vi "Create Arm Constants.vi"(1 "error in":errorcluster, 2 "localConstantSpreadSheet":string[][](array[string]), 3 "robotID":string) -> (0 "error out":errorcluster)   [LabVIEW 2020]
uses:
  2023 Robot Global Data.vi
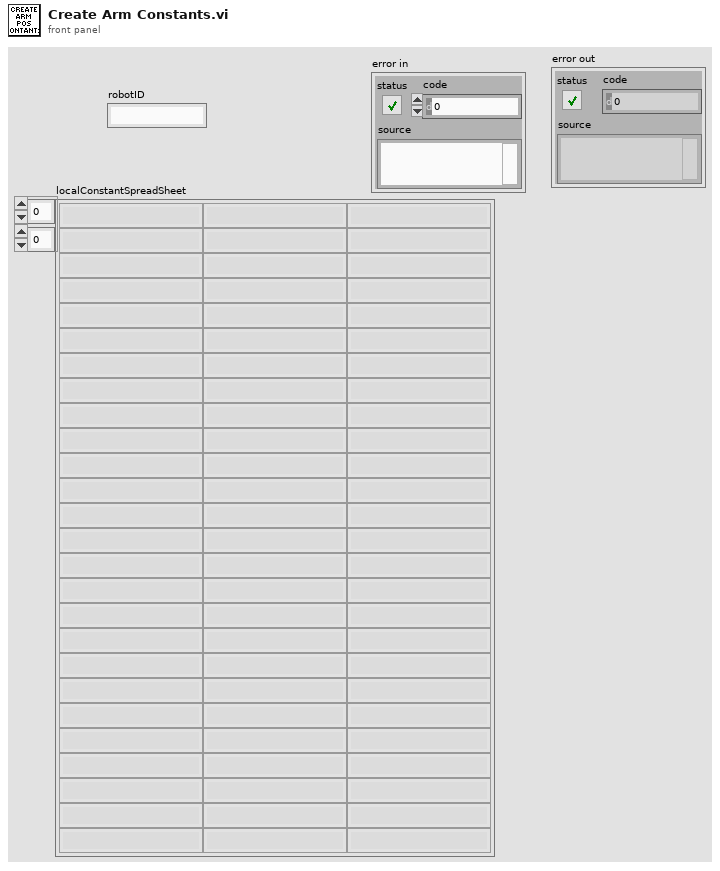
[diagram p1: front panel]
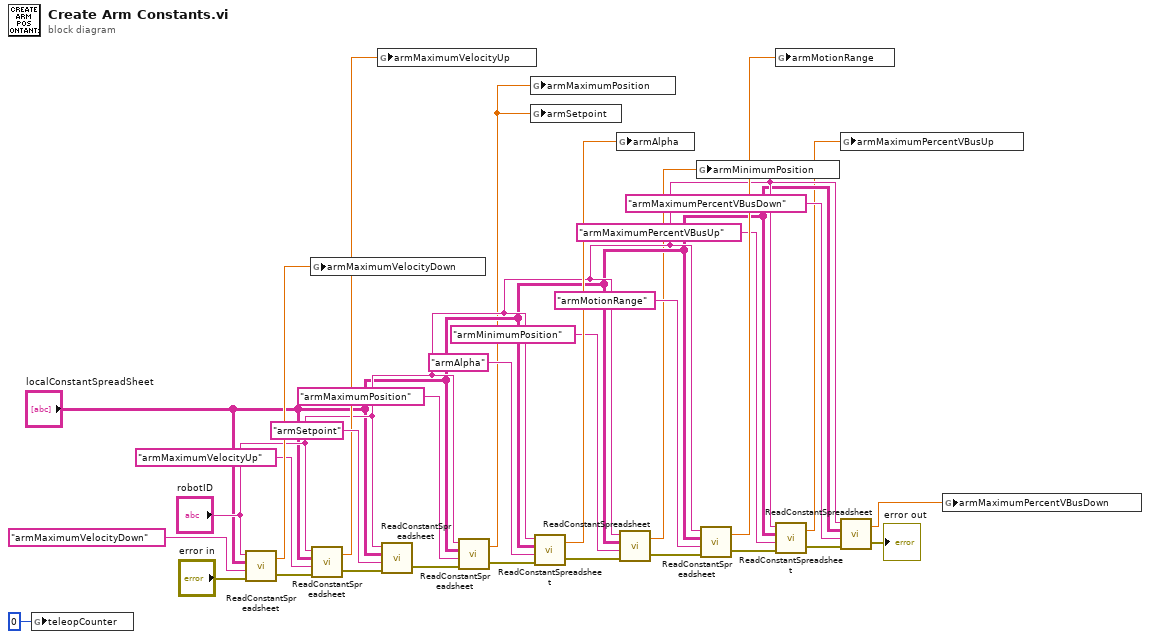
[diagram p0: block diagram]
diagram:
  n1 = global write "2023 Robot Global Data.vi" "teleopCounter"(0 ("teleopCounter")) -> ()
  n2 = call "ReadConstantSpreadsheet.vi"("error in"="error in", "Constant"="armMaximumVelocityDown", "2023ConstantSpreadSheet"="localConstantSpreadSheet", "Robot ID"="robotID") -> ("error out"=w13:errorcluster, "Constant Value"=w28:dbl)
  n3 = global write "2023 Robot Global Data.vi" "armMaximumVelocityDown"(w28) -> ()
  n4 = call "ReadConstantSpreadsheet.vi"("error in"=w13, "Constant"="armMaximumVelocityUp", "2023ConstantSpreadSheet"="localConstantSpreadSheet", "Robot ID"="robotID") -> ("error out"=w12:errorcluster, "Constant Value"=w11:dbl)
  n5 = global write "2023 Robot Global Data.vi" "armMaximumVelocityUp"(w11) -> ()
  n6 = call "ReadConstantSpreadsheet.vi"("error in"=w12, "Constant"="armSetpoint", "2023ConstantSpreadSheet"="localConstantSpreadSheet", "Robot ID"="robotID") -> ("error out"=w5:errorcluster)  [unwired: 1 out]
  n7 = call "ReadConstantSpreadsheet.vi"("error in"=w5, "Constant"="armMaximumPosition", "2023ConstantSpreadSheet"="localConstantSpreadSheet", "Robot ID"="robotID") -> ("error out"=w20:errorcluster, "Constant Value"=w2:dbl)
  n8 = global write "2023 Robot Global Data.vi" "armMaximumPosition"(w2) -> ()
  n9 = global write "2023 Robot Global Data.vi" "armSetpoint"(w2) -> ()
  n10 = call "ReadConstantSpreadsheet.vi"("error in"=w20, "Constant"="armAlpha", "2023ConstantSpreadSheet"="localConstantSpreadSheet", "Robot ID"="robotID") -> ("error out"=w19:errorcluster, "Constant Value"=w26:dbl)
  n11 = global write "2023 Robot Global Data.vi" "armAlpha"(w26) -> ()
  n12 = call "ReadConstantSpreadsheet.vi"("error in"=w19, "Constant"="armMinimumPosition", "2023ConstantSpreadSheet"="localConstantSpreadSheet", "Robot ID"="robotID") -> ("error out"=w18:errorcluster, "Constant Value"=w4:dbl)
  n13 = global write "2023 Robot Global Data.vi" "armMinimumPosition"(w4) -> ()
  n14 = call "ReadConstantSpreadsheet.vi"("error in"=w18, "Constant"="armMotionRange", "2023ConstantSpreadSheet"="localConstantSpreadSheet", "Robot ID"="robotID") -> ("error out"=w10:errorcluster, "Constant Value"=w30:dbl)
  n15 = global write "2023 Robot Global Data.vi" "armMotionRange"(w30) -> ()
  n16 = call "ReadConstantSpreadsheet.vi"("error in"=w10, "Constant"="armMaximumPercentVBusUp", "2023ConstantSpreadSheet"="localConstantSpreadSheet", "Robot ID"="robotID") -> ("error out"=w9:errorcluster, "Constant Value"=w3:dbl)
  n17 = global write "2023 Robot Global Data.vi" "armMaximumPercentVBusUp"(w3) -> ()
  n18 = call "ReadConstantSpreadsheet.vi"("error in"=w9, "Constant"="armMaximumPercentVBusDown", "2023ConstantSpreadSheet"="localConstantSpreadSheet", "Robot ID"="robotID") -> ("error out"=→"error out":errorcluster, "Constant Value"=w17:dbl)
  n19 = global write "2023 Robot Global Data.vi" "armMaximumPercentVBusDown"(w17) -> ()
